vi "Generate Scripting Config Test Data.vi"() -> (3 "Assert Scripting Configuration":T1)   [LabVIEW 2016, in "Create New Assert Tester.lvclass"]
doc: "Generates a set of test data to be used for various tests of scripting functions within the Assert API quick drop and right click framework code"
uses:
  Create New Assert Tester.lvclass
  Plugins/Utility/Assert Scripting Configuration.ctl
  <vilib>/Utility/Data Type/Type Definitions/Data Type.ctl
  <vilib>/Utility/Data Type/NI_Data Type.lvlib
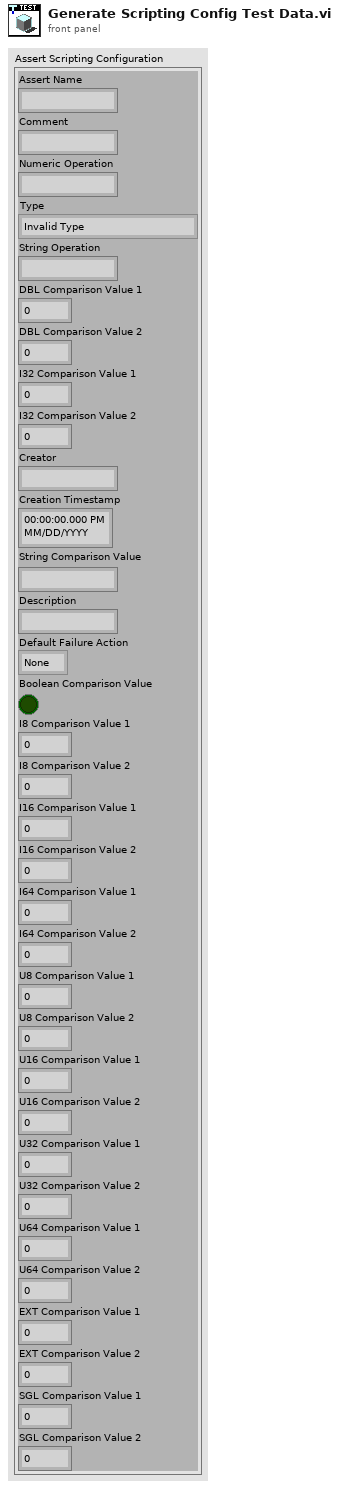
[diagram p1: front panel]
types:
  T1 = typedef "Assert Scripting Configuration.ctl" = cluster{"Assert Name":string, "Comment":string, "Numeric Operation":string, "Type":T2, "String Operation":string, "DBL Comparison Value 1":dbl, "DBL Comparison Value 2":dbl, "I32 Comparison Value 1":i32, "I32 Comparison Value 2":i32, "Creator":string, "Creation Timestamp":timestamp, "String Comparison Value":string, "Description":string, "Default Failure Action":enum16{"None", "Log To File", "Pause Execution", "Abort Execution"}, "Boolean Comparison Value":bool, "I8 Comparison Value 1":i8, "I8 Comparison Value 2":i8, "I16 Comparison Value 1":i16, "I16 Comparison Value 2":i16, "I64 Comparison Value 1":i64, "I64 Comparison Value 2":i64, "U8 Comparison Value 1":u8, "U8 Comparison Value 2":u8, "U16 Comparison Value 1":u16, "U16 Comparison Value 2":u16, "U32 Comparison Value 1":u32, "U32 Comparison Value 2":u32, "U64 Comparison Value 1":u64, "U64 Comparison Value 2":u64, "EXT Comparison Value 1":ext, "EXT Comparison Value 2":ext, "SGL Comparison Value 1":sgl, "SGL Comparison Value 2":sgl}
  T2 = typedef "NI_Data Type.lvlib/Data Type.ctl" = enum8{"Invalid Type", "Void", "I8", "I16", "I32", "I64", "U8", "U16", "U32", "U64", "Single Float", "Double Float", "Extended Float", "Single Complex", "Double Complex", "Extended Complex", "Enum U8", "Enum U16", "Enum U32", "Enum U64", "Single Float With Unit", "Double Float With Unit", "Extended Float With Unit", "Single Complex with Unit", "Double Complex with Unit", "Extended Complex with Unit", "Boolean", "String", "Path", "Picture", "Tag", "Array", "Cluster", "Variant", "LV Variant", "Waveform", "Timestamp", "Digital Waveform", "Digital Data", "ExpressData", "Refnum", "External Data", "VI", "Poly VI", "LabVIEW Class Instance", "Fixed Point"}
  T3 = enum16{"None", "Log To File", "Pause Execution", "Abort Execution"}
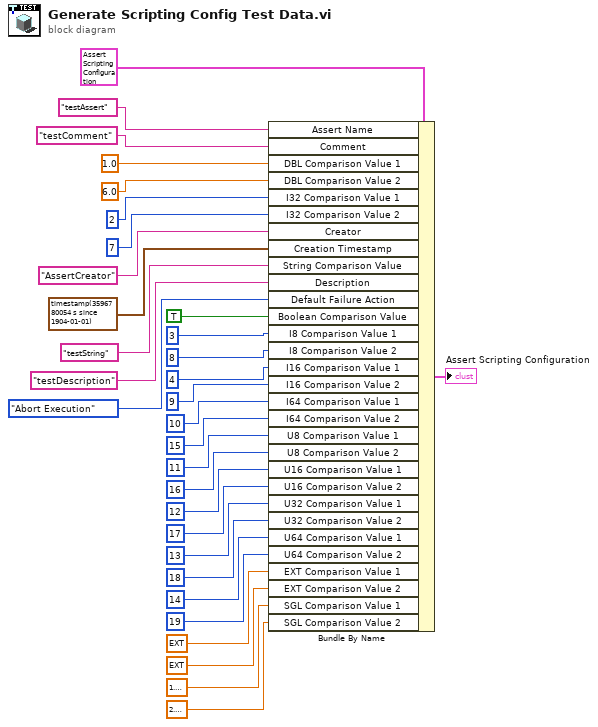
[diagram p0: block diagram]
diagram:
  n1 = Bundle By Name(cluster=T1 {"Assert Name"="", "Comment"="", "Numeric Operation"="", "Type"=enum."Double Float", "String Operation"="", "DBL Comparison Value 1"=0.0, "DBL Comparison Value 2"=0.0, "I32 Comparison Value 1"=0, "I32 Comparison Value 2"=0, "Creator"="", "Creation Timestamp"=timestamp(0 s since 1904-01-01), "String Comparison Value"="", "Description"="", "Default Failure Action"=enum."None", "Boolean Comparison Value"=FALSE, "I8 Comparison Value 1"=0, "I8 Comparison Value 2"=0, "I16 Comparison Value 1"=0, "I16 Comparison Value 2"=0, "I64 Comparison Value 1"=0, "I64 Comparison Value 2"=0, "U8 Comparison Value 1"=0, "U8 Comparison Value 2"=0, "U16 Comparison Value 1"=0, "U16 Comparison Value 2"=0, "U32 Comparison Value 1"=0, "U32 Comparison Value 2"=0, "U64 Comparison Value 1"=0, "U64 Comparison Value 2"=0, "EXT Comparison Value 1"=0.0, "EXT Comparison Value 2"=0.0, "SGL Comparison Value 1"=0.0, "SGL Comparison Value 2"=0.0} ("Assert Scripting Configuration"), "Assert Name"="testAssert", "Comment"="testComment", "DBL Comparison Value 1"=1.0, "DBL Comparison Value 2"=6.0, "I32 Comparison Value 1"=2, "I32 Comparison Value 2"=7, "Creator"="AssertCreator", "Creation Timestamp"=timestamp(3596780054.240864 s since 1904-01-01), "String Comparison Value"="testString", "Description"="testDescription", "Default Failure Action"=T3."Abort Execution", "Boolean Comparison Value"=TRUE, "I8 Comparison Value 1"=i8 3, "I8 Comparison Value 2"=i8 8, "I16 Comparison Value 1"=i16 4, "I16 Comparison Value 2"=i16 9, "I64 Comparison Value 1"=i64 10, "I64 Comparison Value 2"=i64 15, "U8 Comparison Value 1"=u8 11, "U8 Comparison Value 2"=u8 16, "U16 Comparison Value 1"=u16 12, "U16 Comparison Value 2"=u16 17, "U32 Comparison Value 1"=u32 13, "U32 Comparison Value 2"=u32 18, "U64 Comparison Value 1"=u64 14, "U64 Comparison Value 2"=u64 19, "EXT Comparison Value 1"=ext 1.5, "EXT Comparison Value 2"=ext 2.5, "SGL Comparison Value 1"=sgl 1.9, "SGL Comparison Value 2"=sgl 2.7) -> (→"Assert Scripting Configuration":T1)
